vi "Format Sweep XY.vi"(6 "Sweeping?":bool, 7 "ChassisSerialNumber":u32, 8 "REF Channel":i32, 9 "Channel":i32, 10 "Y":waveform(dbl), 11 "X":waveform(dbl)) -> (2 "Times":timestamp[](array[timestamp]), 3 "Array":T1[](array[typedef]))   [LabVIEW 2019, in "Instrument.Lockin.lvlib" / "Instrument.Lockin.lvclass"]
uses:
  Instrument.Lockin.lvclass
  Typedefs/Lockin.LogSweepXY--Cluster.ctl
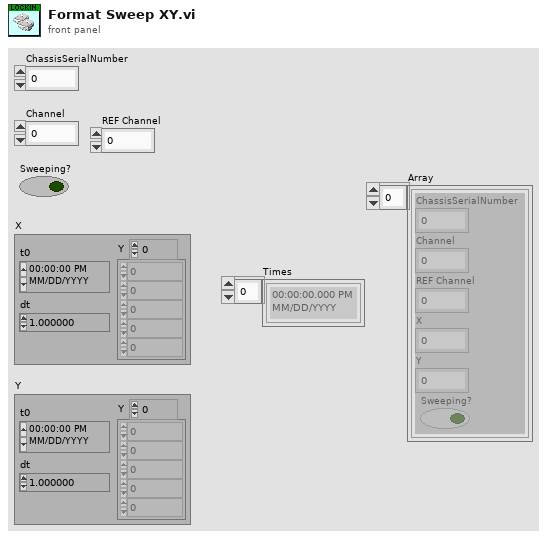
[diagram p1: front panel]
types:
  T1 = typedef "Instrument.Lockin.lvlib/Instrument.Lockin.lvclass/Lockin.LogSweepXY--Cluster.ctl" = cluster{"ChassisSerialNumber":u32, "Channel":i32, "REF Channel":i32, "X":dbl, "Y":dbl, "Sweeping?":bool}
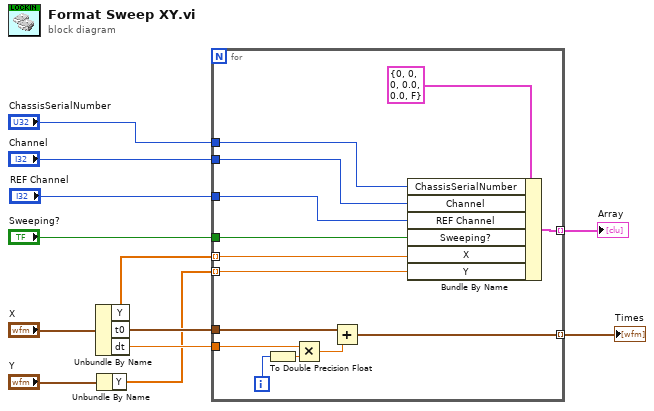
[diagram p0: block diagram]
diagram:
  n1 = Unbundle By Name("X") -> ("Y"=w7:dbl[], "t0"=w5:timestamp, "dt"=w6:dbl)
  n2 = Unbundle By Name("Y") -> ("Y"=w2:dbl[])
  n3 = for {
    tunnel: w5 -> [w22]
    tunnel: w6 -> [w26]
    tunnel: [w21] -> w12 mode=indexing
    tunnel: w7 -> [w17] mode=indexing
    tunnel: "ChassisSerialNumber" -> [w14]
    tunnel: "Channel" -> [w15]
    tunnel: "Sweeping?" -> [w19]
    tunnel: [w18] -> w4 mode=indexing
    tunnel: w2 -> [w16] mode=indexing
    tunnel: "REF Channel" -> [w13]
    i -> [w25]
    n4 = To Double Precision Float(number=w25) -> (double precision float=w24:dbl)
    n5 = Multiply(x=w26, y=w24) -> (x*y=w23:dbl)
    n6 = Add(x=w22, y=w23) -> (x+y=w21:timestamp)
    n7 = Bundle By Name(cluster=T1 {"ChassisSerialNumber"=0, "Channel"=0, "REF Channel"=0, "X"=0.0, "Y"=0.0, "Sweeping?"=FALSE}, "ChassisSerialNumber"=w14, "Channel"=w15, "REF Channel"=w13, "Sweeping?"=w19, "X"=w17, "Y"=w16) -> (w18:T1)
  }
  "Times" <- w12
  "Array" <- w4
